vi "DC_CNTRL_gen_max_pot_array.vi"(0 "Handle":u64, 1 "Number of supplies in box":i32, 3 "Box Number":u16(ring), 11 "error in (no error)":errorcluster) -> (4 "Handle out":u64, 13 "Max Range Aray":dbl[](array[numeric]), 15 "error out":errorcluster)   [LabVIEW 2019]
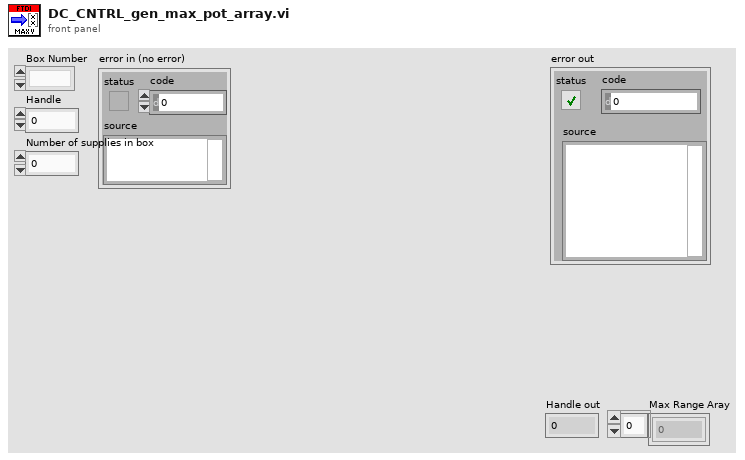
[diagram p1: front panel]
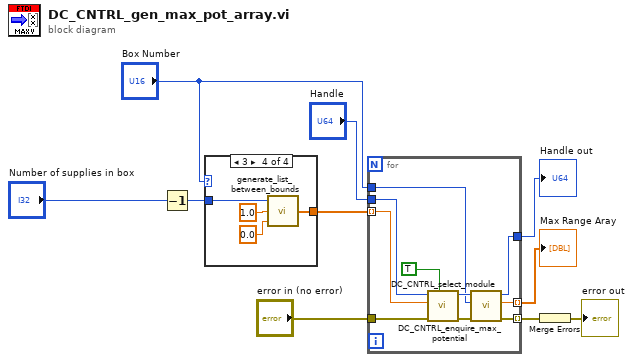
[diagram p0: block diagram]
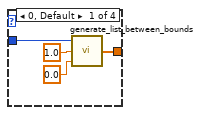
[diagram p2: hidden frame]
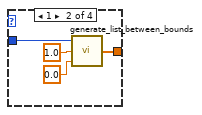
[diagram p3: hidden frame]
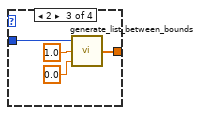
[diagram p4: hidden frame]
diagram:
  n1 = Decrement(x="Number of supplies in box") -> (x-1=w2:i32)
  n2 = case shown="3" "Box Number" {
    tunnel: [w12 w16 w20 w24] -> w10
    tunnel: w2 -> [w11 w15 w19 w23]
    frame 0, Default {
      n3 = call "generate_list_between_bounds.vi"("Upper bound"=w11, "Step size"=1.0, "Lower bound"=0.0) -> ("Array"=w12:dbl[])  [unwired: 2 in]
    }
    frame 1 {
      n4 = call "generate_list_between_bounds.vi"("Upper bound"=w15, "Step size"=1.0, "Lower bound"=0.0) -> ("Array"=w16:dbl[])  [unwired: 2 in]
    }
    frame 2 {
      n5 = call "generate_list_between_bounds.vi"("Upper bound"=w19, "Step size"=1.0, "Lower bound"=0.0) -> ("Array"=w20:dbl[])  [unwired: 2 in]
    }
    frame 3 {
      n6 = call "generate_list_between_bounds.vi"("Upper bound"=w23, "Step size"=1.0, "Lower bound"=0.0) -> ("Array"=w24:dbl[])  [unwired: 2 in]
    }
  }
  n7 = for {
    tunnel: w10 -> [w32] mode=indexing
    tunnel: "Handle" -> [w36]
    tunnel: "error in (no error)" -> [w35]
    tunnel: [w31] -> w5
    tunnel: [w30] -> w7 mode=indexing
    tunnel: [w29] -> w4 mode=indexing
    tunnel: "Box Number" -> [w27]
    n8 = call "DC_CNTRL_select_module.vi"("Read Answer?"=TRUE, "error in (no error)"=w35, "Module number"=w32, "Handle"=w36) -> ("error out"=w33:errorcluster, "Handle out"=w34:u64)  [unwired: 6 in]
    n9 = call "DC_CNTRL_enquire_max_potential.vi"("error in (no error)"=w33, "Box Number"=w27, "Handle"=w34) -> ("error out"=w30:errorcluster, "Max Value"=w29:dbl, "Handle out"=w31:u64)  [unwired: 6 in]
  }
  "Handle out" <- w5
  "Max Range Aray" <- w4
  n10 = Merge Errors(w7) -> (→"error out":errorcluster)
